vi "Read configuration.vi"(11 "lvlibretls configurable context in":refnum<class "lvlibretls configurable context.lvclass">) -> (2 "configuration":u64)   [LabVIEW 2016, in "lvlibretls configurable context.lvclass"]
uses:
  lvlibretls configurable context.lvclass
  lvlibretls configurable context.lvclass/lvlibretls configurable context.ctl
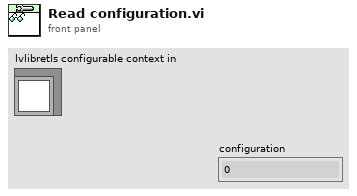
[diagram p1: front panel]
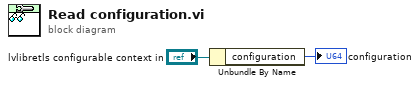
[diagram p0: block diagram]
diagram:
  n1 = Unbundle By Name("lvlibretls configurable context in") -> ("configuration"=→"configuration":u64)
